vi "Write JSON Config.vi"(6 "Pretty Print?":bool, 8 "error in (no error)":errorcluster, 11 "ConvertTo_U64 in":refnum<class "ConvertTo_U64.lvclass">) -> (0 "error out":errorcluster, 2 "JSON":string, 3 "ConvertTo_U64 out":refnum<class "ConvertTo_U64.lvclass">)   [LabVIEW 2021, in "ConvertTo_U64.lvclass"]
uses:
  ConvertTo_U64.lvclass
  Abs_Types/U64 Integer/Abs_U64 Integer.lvclass
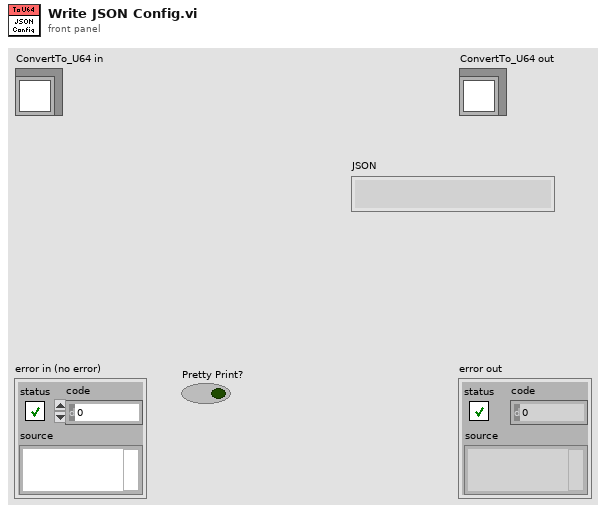
[diagram p1: front panel]
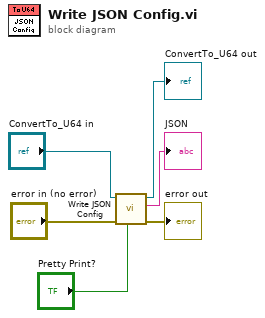
[diagram p0: block diagram]
diagram:
  n1 = call-parent "Write JSON Config.vi"("Pretty Print?"="Pretty Print?", "error in (no error)"="error in (no error)", "Abs_Type in"="ConvertTo_U64 in") -> ("error out"=→"error out":errorcluster, "JSON"=→"JSON":string, "Abs_Type out"=→"ConvertTo_U64 out":refnum<class "ConvertTo_U64.lvclass">)  [unwired: 6 in]
